vi "ForceDataChange.vi"(2 "index":i32, 3 "data":string="\"§¶C54ÍÀì6#D\u000b\u00033Ã\u0014ð©À\u0002°B\u0000\u0000\u0000\u0000\u0000\u0000\u0000\u0000\u0006\u0000\u0000\u0000\u0000\u0000\u0010\u0000") -> (0 "数值":sgl, 1 "out":sgl[](array[numeric]))   [LabVIEW 2018]
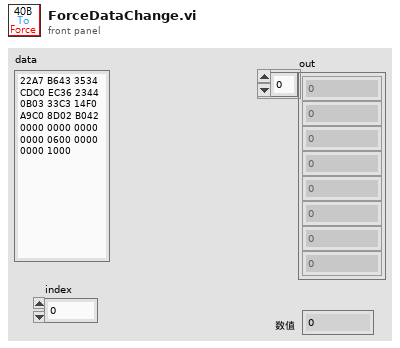
[diagram p1: front panel]
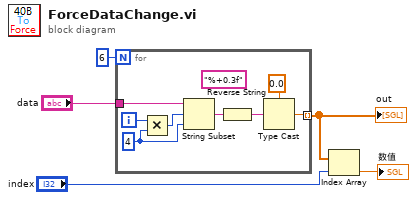
[diagram p0: block diagram]
diagram:
  n1 = for {
    N: 6 -> [_]
    tunnel: "data" -> [w13]
    tunnel: [w6] -> w3 mode=indexing
    i -> [w8]
    (unwired) "%+0.3f"
    w10 = 4
    n2 = Multiply(x=w8, y=w10) -> (x*y=w12:i32)
    n3 = String Subset(string=w13, offset (0)=w12, length (rest)=w10) -> (substring=w11:string)
    n4 = Reverse String(1:w11) -> (0:w9:string)
    n5 = Type Cast(type=sgl 0.0, x=w9) -> (*(type *) &x=w6:sgl)
  }
  "out" <- w3
  n6 = Index Array(array=w3, index="index") -> (element=→"数值":sgl)
